vi "Design a Floating-Point Multirate Filter Part 1.vi"   [LabVIEW 2023]
doc: "Part 1 of the Designing a Floating-Point Multirate Filter tutorial."
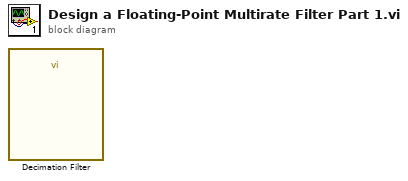
[diagram p0: block diagram]
diagram:
  n1 = call "Decimation Filter"() -> ()  [unwired: 10 in, 2 out]
